vi "Recursive Folder List.vi"(4 "Folders to Exclude":string[](array[string]), 6 "pattern":string, 8 "error in (no error)":errorcluster, 9 "Continue Recursing on Error? (F)":bool, 11 "Folder Path":path) -> (0 "error out":errorcluster, 1 "Number of Folders":i32, 2 "All Folders":path[](array[path]), 3 "Folder Path out":path)   [LabVIEW 2017]
doc: "Recursively lists every folder under Folder Path whose name matches pattern, skipping the names listed in Folders to Exclude."
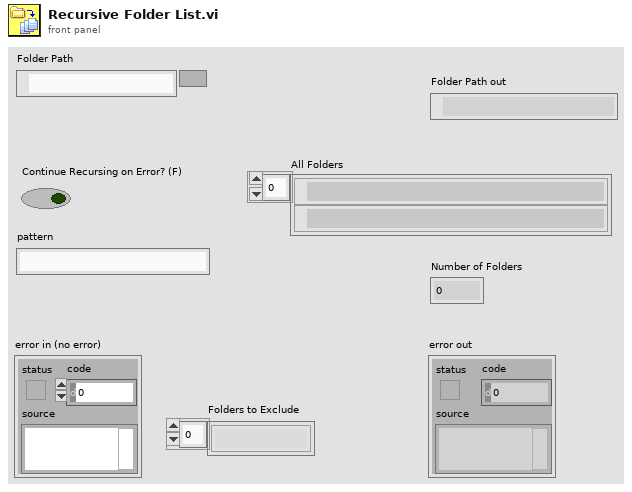
[diagram p1: front panel]
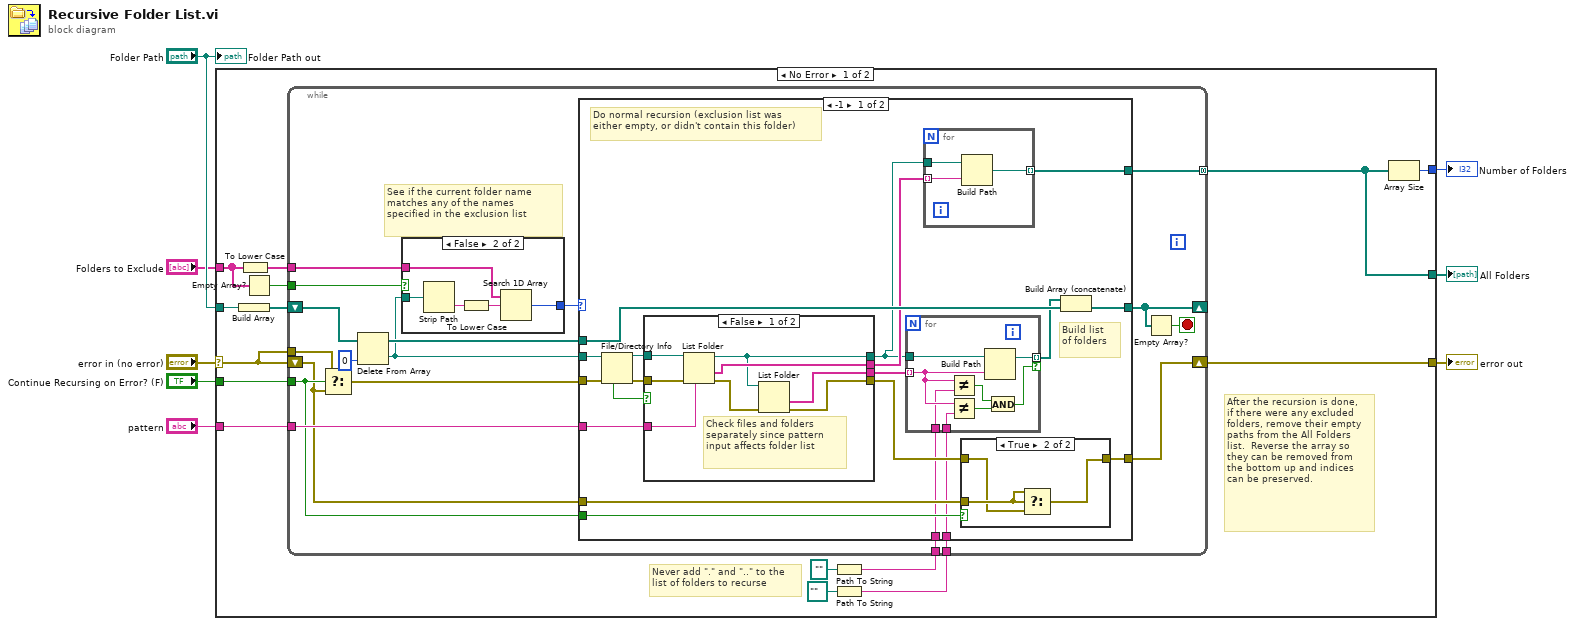
[diagram p0: block diagram]
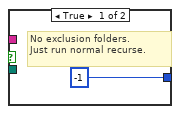
[diagram p2: hidden frame]
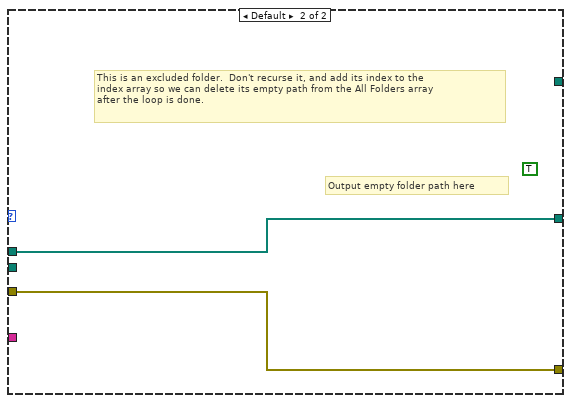
[diagram p5: hidden frame]
diagram:
  n1 = case shown="No Error" "error in (no error)" {
    selector: "error in (no error)" -> [w17 w94]
    tunnel: "Folder Path" -> [w23 _]
    tunnel: [w19 _] -> w8
    tunnel: [w20 w94] -> w7
    tunnel: "pattern" -> [w21 _]
    tunnel: "Continue Recursing on Error? (F)" -> [w18 _]
    tunnel: "Folders to Exclude" -> [w15 _]
    tunnel: [w9 _] -> w1
    frame No Error {
      # "Never add \".\" and \"..\" to the list of folders to recurse"
      # "After the recursion is done,\nif there were any excluded\nfolders, remove their empty\npaths from the All Folders\nlist.  Reverse the array so\nthey can be removed from\nthe bottom up and indices\ncan be preserved."
      n2 = Build Array(w23) -> (w22:path[])
      n3 = To Lower Case(string=w15) -> (all lower case string=w16:string[])
      n4 = Empty Array?(array=w15) -> (empty?=w14:bool)
      n5 = Path To String(path=path "") -> (string=w11:string)
      n6 = Path To String(path=path "..") -> (string=w10:string)
      n7 = while {
        shift-left: w22 -> [w41]
        shift-right: [w39] -> _
        shift-right: [w33] -> w20
        shift-left: w17 -> [w32]
        tunnel: w21 -> [w40]
        tunnel: w18 -> [w34]
        tunnel: w17 -> [w35]
        tunnel: w16 -> [w29]
        tunnel: w14 -> [w30]
        tunnel: w11 -> [w26]
        tunnel: w10 -> [w25]
        tunnel: [w24] -> w9 mode=concatenating
        stop <- w38 stop-if-true
        # "See if the current folder name\nmatches any of the names\nspecified in the exclusion list"
        n8 = Select(t=w35, s=w34, f=w32) -> (s? t:f=w36:errorcluster)
        n9 = Delete From Array(array=w41, index=0) -> (deleted portion=w28:path, array with subset deleted=w31:path[])  [unwired: 1 in]
        n10 = case shown="False" w30 {
          tunnel: w29 -> [_ w44]
          tunnel: w28 -> [_ w47]
          tunnel: [-1 ("index of element") w43] -> w27
          frame True {
            # "No exclusion folders.\nJust run normal recurse."
          }
          frame False {
            n11 = Strip Path(path=w47) -> (name=w46:string)  [unwired: 1 out]
            n12 = To Lower Case(string=w46) -> (all lower case string=w45:string)
            n13 = Search 1D Array(1D array=w44, element=w45) -> (index of element=w43:i32)  [unwired: 1 out]
          }
        }
        n14 = case shown="-1" w27 {
          tunnel: w40 -> [w66 _]
          tunnel: [w64 w93] -> w39
          tunnel: w28 -> [w54 _]
          tunnel: w36 -> [w60 w92]
          tunnel: w34 -> [w58 _]
          tunnel: [w57 w92] -> w33
          tunnel: w32 -> [w56 _]
          tunnel: w31 -> [w55 w93]
          tunnel: w26 -> [w52 _]
          tunnel: w25 -> [w51 _]
          tunnel: [w48 _] -> w24
          frame -1 {
            # "Build list\nof folders"
            # "Do normal recursion (exclusion list was\neither empty, or didn't contain this folder)"
            n15 = File/Directory Info(path=w54, error in=w60) -> (path out=w62:path, error out=w63:errorcluster, shortcut=w61:bool)  [unwired: 4 out]
            n16 = case shown="False" w61 {
              tunnel: [w85 _] -> w50
              tunnel: [w84 w87] -> w49
              tunnel: [w83 w86] -> w59
              tunnel: w66 -> [w82 _]
              tunnel: [w78 _] -> w65
              tunnel: w63 -> [w81 w86]
              tunnel: w62 -> [w80 w87]
              frame False {
                # "Check files and folders\nseparately since pattern\ninput affects folder list"
                n17 = List Folder(path=w80, pattern=w82, error in=w81) -> (path out=w84:path, folder names=w85:string[], error out=w79:errorcluster)  [unwired: 2 out]
                n18 = List Folder(path=w84, error in=w79) -> (folder names=w78:string[], error out=w83:errorcluster)  [unwired: 4 out]
              }
              frame True {
                # "Do not attempt to recurse the contents of folder shortcuts"
              }
            }
            n19 = for {
              tunnel: w49 -> [w77]
              tunnel: [w76] -> w53 mode=indexing if=w75
              tunnel: w65 -> [w74] mode=indexing
              tunnel: w52 -> [w73]
              tunnel: w51 -> [w72]
              n20 = Not Equal?(x=w74, y=w73) -> (x != y?=w70:bool)
              n21 = Not Equal?(x=w74, y=w72) -> (x != y?=w71:bool)
              n22 = Build Path(base path=w77, name or relative path=w74) -> (appended path=w76:path)
              n23 = And(x=w70, y=w71) -> (x .and. y?=w75:bool)
            }
            n24 = for {
              tunnel: w50 -> [w69] mode=indexing
              tunnel: w49 -> [w68]
              tunnel: [w67] -> w48 mode=indexing
              n25 = Build Path(base path=w68, name or relative path=w69) -> (appended path=w67:path)
            }
            n26 = case shown="True" w58 {
              tunnel: w59 -> [w88 w90]
              tunnel: [w88 w89] -> w57
              tunnel: w56 -> [_ w91]
              frame False {
              }
              frame True {
                n27 = Select(t=w91, s=w91, f=w90) -> (s? t:f=w89:errorcluster)
              }
            }
            n28 = Build Array (concatenate)(w53, w55) -> (w64:path[])
          }
          frame Default {
            (unwired) TRUE
            # "Output empty folder path here"
            # "This is an excluded folder.  Don't recurse it, and add its index to the\nindex array so we can delete its empty path from the All Folders array\nafter the loop is done."
          }
        }
        n29 = Empty Array?(array=w39) -> (empty?=w38:bool)
      }
      n30 = Array Size(array=w9) -> (size(s)=w19:i32)
    }
    frame Error {
    }
  }
  "Number of Folders" <- w8
  "error out" <- w7
  "All Folders" <- w1
  "Folder Path out" <- "Folder Path"
